vi "Matrix Quick Invert.vi"(11 "Matrix":sgl[][](array[numeric])) -> (3 "Matrix Inverted":sgl[][](array[numeric]))   [LabVIEW 2020, in "3D.lvlib"]
uses:
  3D.lvlib
panel:
  # "This maths is only valid for Translation / Rotation matrices!"
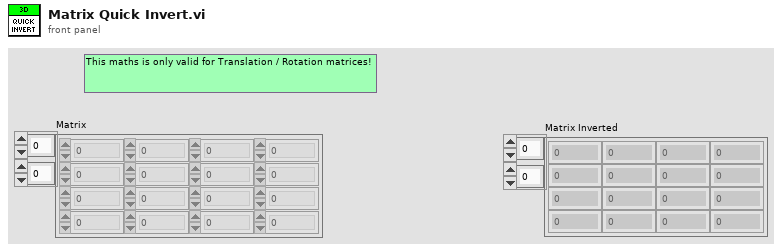
[diagram p1: front panel]
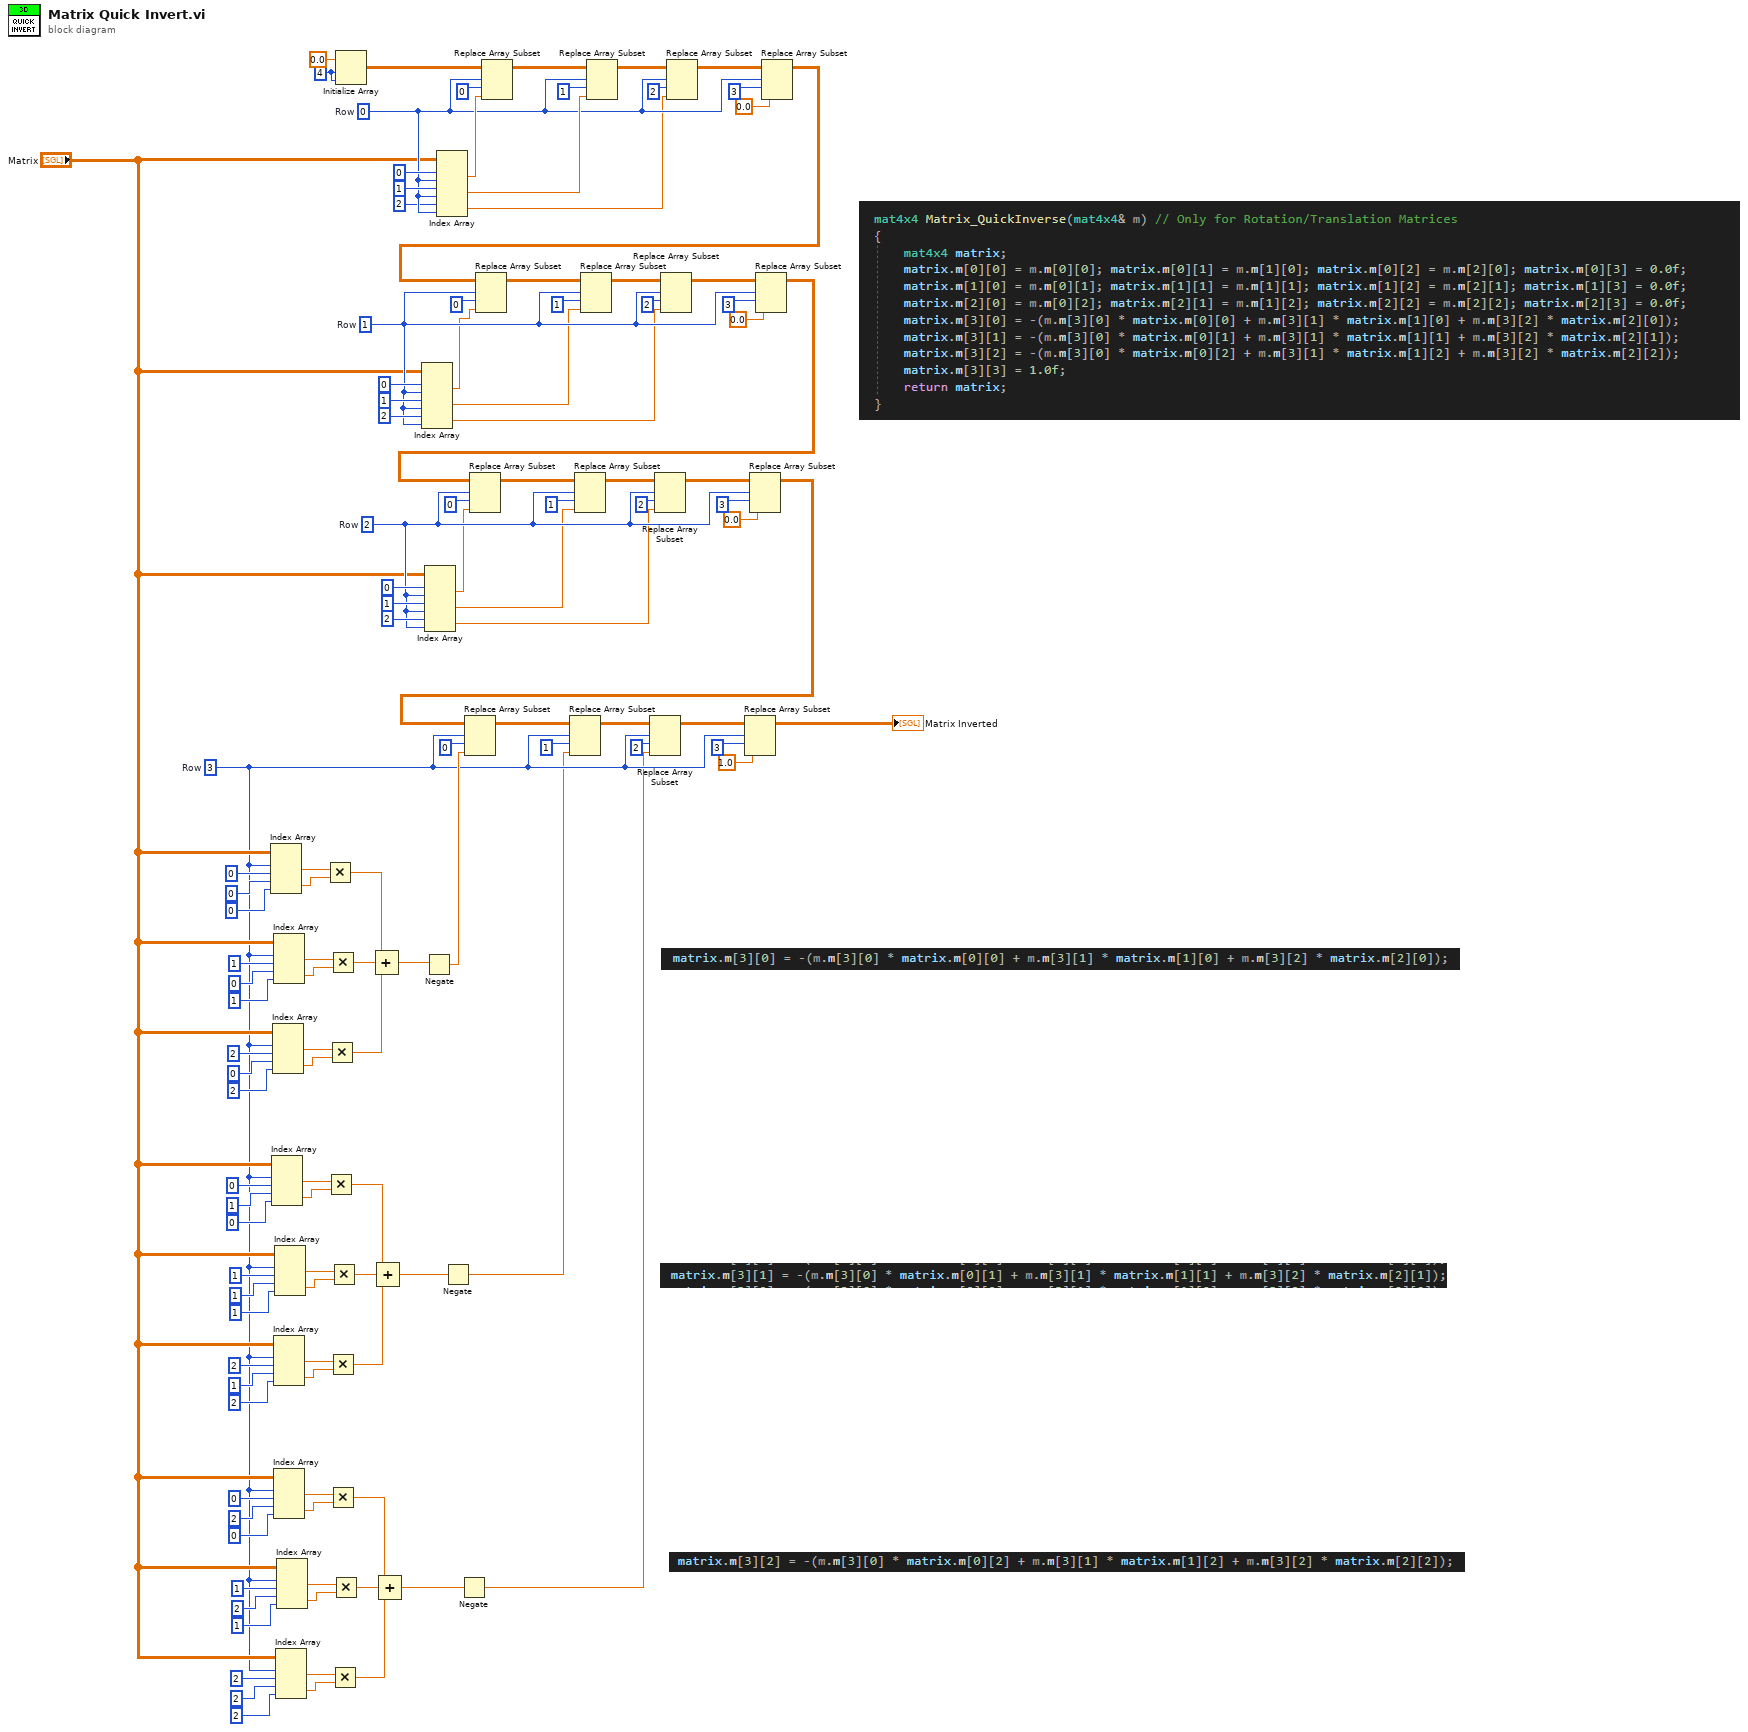
[diagram p0: block diagram]
diagram:
  w5 = 3  # Row
  w67 = 2  # Row
  w75 = 1  # Row
  w81 = 0  # Row
  w121 = 4 ("dimension size")
  n1 = Index Array(array="Matrix", index (row) #1=w5, index (col) #1=0 ("disabled index (col)"), index (row) #2=0 ("index (row)"), index (col) #2=0 ("index (row)")) -> (element #1=w59:sgl, element #2=w58:sgl)
  n2 = Index Array(array="Matrix", index (row) #1=w5, index (col) #1=0 ("disabled index (col)"), index (row) #2=1 ("index (row)"), index (col) #2=0 ("index (row)")) -> (element #1=w28:sgl, element #2=w29:sgl)
  n3 = Index Array(array="Matrix", index (row) #1=w5, index (col) #1=2 ("disabled index (col)"), index (row) #2=0 ("index (row)"), index (col) #2=2 ("index (row)")) -> (element #1=w49:sgl, element #2=w48:sgl)
  n4 = Index Array(array="Matrix", index (row) #1=w5, index (col) #1=1 ("disabled index (col)"), index (row) #2=0 ("index (row)"), index (col) #2=1 ("index (row)")) -> (element #1=w56:sgl, element #2=w57:sgl)
  n5 = Index Array(array="Matrix", index (row) #1=w5, index (col) #1=2 ("disabled index (col)"), index (row) #2=1 ("index (row)"), index (col) #2=2 ("index (row)")) -> (element #1=w38:sgl, element #2=w39:sgl)
  n6 = Index Array(array="Matrix", index (row) #1=w5, index (col) #1=0 ("disabled index (col)"), index (row) #2=2 ("index (row)"), index (col) #2=0 ("index (row)")) -> (element #1=w21:sgl, element #2=w20:sgl)
  n7 = Index Array(array="Matrix", index (row) #1=w5, index (col) #1=1 ("disabled index (col)"), index (row) #2=1 ("index (row)"), index (col) #2=1 ("index (row)")) -> (element #1=w31:sgl, element #2=w30:sgl)
  n8 = Index Array(array="Matrix", index (row) #1=w5, index (col) #1=2 ("disabled index (col)"), index (row) #2=2 ("index (row)"), index (col) #2=2 ("index (row)")) -> (element #1=w11:sgl, element #2=w10:sgl)
  n9 = Index Array(array="Matrix", index (row) #1=w5, index (col) #1=1 ("disabled index (col)"), index (row) #2=2 ("index (row)"), index (col) #2=1 ("index (row)")) -> (element #1=w18:sgl, element #2=w19:sgl)
  n10 = Multiply(x=w59, y=w58) -> (x*y=w47:sgl)
  n11 = Multiply(x=w28, y=w29) -> (x*y=w40:sgl)
  n12 = Multiply(x=w49, y=w48) -> (x*y=w45:sgl)
  n13 = Multiply(x=w56, y=w57) -> (x*y=w46:sgl)
  n14 = Multiply(x=w38, y=w39) -> (x*y=w42:sgl)
  n15 = Multiply(x=w21, y=w20) -> (x*y=w9:sgl)
  n16 = Multiply(x=w31, y=w30) -> (x*y=w41:sgl)
  n17 = Multiply(x=w11, y=w10) -> (x*y=w7:sgl)
  n18 = Multiply(x=w18, y=w19) -> (x*y=w8:sgl)
  n19 = Initialize Array(sgl 0.0 ("element"), w121, w121) -> (w120:sgl[][])
  n20 = Compound Arithmetic op=ADD(w47, w46, w45) -> (w44:sgl)
  n21 = Compound Arithmetic op=ADD(w40, w41, w42) -> (w4:sgl)
  n22 = Compound Arithmetic op=ADD(w9, w8, w7) -> (w2:sgl)
  n23 = Index Array(array="Matrix", index (row) #1=0 ("index (row)"), index (col) #1=w75, index (row) #2=1 ("disabled index (col)"), index (col) #2=w75, index (row) #3=2 ("disabled index (col)"), index (col) #3=w75) -> (element #1=w74:sgl, element #2=w73:sgl, element #3=w72:sgl)
  n24 = Negate(x=w44) -> (-x=w43:sgl)
  n25 = Index Array(array="Matrix", index (row) #1=0 ("index (row)"), index (col) #1=w67, index (row) #2=1 ("disabled index (col)"), index (col) #2=w67, index (row) #3=2 ("disabled index (col)"), index (col) #3=w67) -> (element #1=w66:sgl, element #2=w65:sgl, element #3=w64:sgl)
  n26 = Index Array(array="Matrix", index (row) #1=0 ("index (row)"), index (col) #1=w81, index (row) #2=1 ("disabled index (col)"), index (col) #2=w81, index (row) #3=2 ("disabled index (col)"), index (col) #3=w81) -> (element #1=w86:sgl, element #2=w83:sgl, element #3=w79:sgl)
  n27 = Negate(x=w4) -> (-x=w3:sgl)
  n28 = Negate(x=w2) -> (-x=w1:sgl)
  n29 = Replace Array Subset(array=w120, new element=w86, index (row)=w81, index (col)=0 ("index (row)")) -> (w117:sgl[][])
  n30 = Replace Array Subset(array=w117, new element=w83, index (row)=w81, index (col)=1 ("index (row)")) -> (w115:sgl[][])
  n31 = Replace Array Subset(array=w115, new element=w79, index (row)=w81, index (col)=2 ("index (row)")) -> (w113:sgl[][])
  n32 = Replace Array Subset(array=w113, new element=sgl 0.0 ("new element/subarray"), index (row)=w81, index (col)=3 ("index (row)")) -> (w105:sgl[][])
  n33 = Replace Array Subset(array=w105, new element=w74, index (row)=w75, index (col)=0 ("index (row)")) -> (w108:sgl[][])
  n34 = Replace Array Subset(array=w108, new element=w73, index (row)=w75, index (col)=1 ("index (row)")) -> (w110:sgl[][])
  n35 = Replace Array Subset(array=w110, new element=w72, index (row)=w75, index (col)=2 ("index (row)")) -> (w112:sgl[][])
  n36 = Replace Array Subset(array=w112, new element=sgl 0.0 ("new element/subarray"), index (row)=w75, index (col)=3 ("index (row)")) -> (w97:sgl[][])
  n37 = Replace Array Subset(array=w97, new element=w66, index (row)=w67, index (col)=0 ("index (row)")) -> (w102:sgl[][])
  n38 = Replace Array Subset(array=w102, new element=w65, index (row)=w67, index (col)=1 ("index (row)")) -> (w100:sgl[][])
  n39 = Replace Array Subset(array=w100, new element=w64, index (row)=w67, index (col)=2 ("index (row)")) -> (w98:sgl[][])
  n40 = Replace Array Subset(array=w98, new element=sgl 0.0 ("new element/subarray"), index (row)=w67, index (col)=3 ("index (row)")) -> (w89:sgl[][])
  n41 = Replace Array Subset(array=w89, new element=w43, index (row)=w5, index (col)=0 ("index (row)")) -> (w92:sgl[][])
  n42 = Replace Array Subset(array=w92, new element=w3, index (row)=w5, index (col)=1 ("index (row)")) -> (w94:sgl[][])
  n43 = Replace Array Subset(array=w94, new element=w1, index (row)=w5, index (col)=2 ("index (row)")) -> (w96:sgl[][])
  n44 = Replace Array Subset(array=w96, new element=sgl 1.0 ("new element/subarray"), index (row)=w5, index (col)=3 ("index (row)")) -> (→"Matrix Inverted":sgl[][])
